vi "3458A Digitizing Process.vi"(8 "error in":errorcluster, 11 "session in":variant) -> (0 "error out":errorcluster, 3 "aux data out":variant)   [LabVIEW 2020, in "3458A Virtual Digitizer.lvlib"]
doc: "3458A digitizing lib: Main digitizing process. The VI is assynchronously executed once for each channel (all in parallel). It is started by calling 'Initiate Digitizing Process'. It then samples and sends the digitized data via queues to main process where the data are collected using 'Fetch Digitized Data'. Configuration of the execution is stored in 'session in' variable, execution control details are in 'session in->proc setup' cluster. Each instance of this VI has ID starting from 0 which identifies to which channel it belongs to."
uses:
  3458A Virtual Digitizer.lvlib
  3458A Digitizer Session.ctl
  3458A Virtual Channel Config.ctl
  Counter/Counter Session.ctl
  Counter/Counter Type.ctl
  AWG/AWG Session.ctl
  AWG/AWG Type.ctl
  AWG/CMI Clock Divider v2/CMI ckd2 Session.ctl
  AWG/CMI Clock Divider v2/CMI ckd2 Source Mode.ctl
  AWG/CMI Clock Divider v2/CMI ckd2 Divisor Mode.ctl
  AWG/CMI Sync V3/CMI Sync V3 session.ctl
  AWG/CMI Sync V3/Configure/CMI Sync V3 Reference Clock Source.ctl
  AWG/CMI Sync V3/Configure/CMI Sync V3 HV input Range.ctl
  AWG/CMI Sync V3/Configure/CMI Sync V3 Trigger Input Level.ctl
  AWG/CMI Sync V3/Configure/CMI Sync V3 Channel 1 Mode.ctl
  AWG/CMI Sync V3/Configure/CMI Sync V3 Channel Output Levels.ctl
  AWG/CMI Sync V3/Configure/CMI Sync V3 Channel 2 Mode.ctl
  AWG/CMI Sync V3/Configure/CMI Sync V3 Channel 3 Mode.ctl
  AWG/CMI Sync V3/Configure/CMI Sync V3 Channel 1 Divisor Entry Mode.ctl
  adc/ADC Trig Config.ctl
  adc/ADC Trig Mode Source.ctl
  adc/ADC Trig Slope.ctl
  adc/ADC Trig Coupling.ctl
  AWG/RaS HMF2500/HMF2500 Config.ctl
  3458A Sync Mode.ctl
  3458A Idn Mode.ctl
  3458A Digitizing Low Levels/Configure/Sampling Mode.ctl
  3458A Digitizing Process Options.ctl
  3458A Data Packet.ctl
  3458A Aux Record Data.ctl
  3458A Digitizing Low Levels/Configure/Level Setup.ctl
  3458A Digitizing Low Levels/Configure/First Sample Trigger.ctl
  3458A Aperture Selection Mode.ctl
  3458A Multiplexing Config.ctl
  Fluke 8588A/F8588A Low Pass Filter.ctl
  Fluke 8588A/F8588A Phase Lock.ctl
  Fluke 8588A/F8588A Coupling.ctl
  3458A Sampling Rate.ctl
  AWG/AWG Clock Setup Mode.ctl
  3458A Sample Rate Mode.ctl
  <vilib>/Utility/error.llb/Error Cluster From Error Code.vi
  <vilib>/ErrorRing/Error Ring.xnode
  Counter/Counter.lvlib
  AWG/AWG.lvlib
  3458A Digitizing Low Levels/3458A Digitizing Low Levels.lvlib
  3458A Basic Driver/3458A Basic Driver.lvlib
  AWG/CMI Sync V3/CMI Sync Unit V3.lvlib
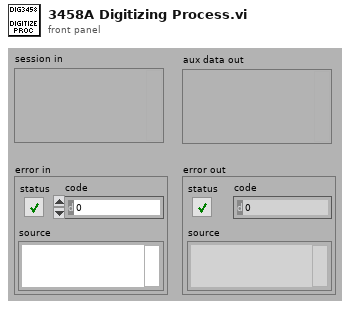
[diagram p1: front panel]
types:
  T1 = typedef "3458A Virtual Digitizer.lvlib/3458A Digitizing Low Levels.lvlib/First Sample Trigger.ctl" = enum16{"AUTO", "EXT", "SYN", "SGL", "HOLD", "LEVEL"}
  T2 = typedef "3458A Virtual Digitizer.lvlib/3458A Data Packet.ctl" = cluster{"data":i32[][], "offset [smpl]":i32, "count [smpl]":i32, "all done?":bool, "sampling?":bool, "queue buffer [%]":dbl, "valid?":bool, "overflow?":bool, "estimate info?":bool}
  T3 = typedef "3458A Virtual Digitizer.lvlib/3458A Digitizer Session.ctl" = cluster{"channels":T4[], "sync unit":T5, "awg unit":T7, "sync mode":T26, "streaming mode":bool, "idn mode":T27, "sampling mode":T28, "sample memory [B]":i32, "proc setup":T29, "sample size [B]":i32, "sample count":i32, "aux data":T31, "ranges [V]":dbl[], "aperture [s]":dbl, "LEVEL trigger":T32, "trigger mode":T1, "measure temp.?":bool, "disp mesages":string[], "shared bus?":bool, "disable display?":bool, "aper mode":T33, "aper rules":dbl[][], "multiplex":T34, "F8588 lpf":T35, "F8588 pll":T36, "F8588 couple":T37, "fs":T38, "fs mode":T40, "init timestamp":timestamp, "last report timestamp":timestamp}
  T4 = typedef "3458A Virtual Digitizer.lvlib/3458A Virtual Channel Config.ctl" = cluster{"VISA":refnum<visa-resource-name>, "Range [Vpk]":dbl, "btn clr":bool, "btn up":bool, "btn down":bool, "F8588":bool, "F8588 guard":bool}
  T5 = typedef "Counter.lvlib/Counter Session.ctl" = cluster{"VISA":refnum<visa-resource-name>, "type":T6}
  T6 = typedef "Counter.lvlib/Counter Type.ctl" = enum16{"Picotest U6200A", "dummy"}
  T7 = typedef "AWG.lvlib/AWG Session.ctl" = cluster{"type":T8, "VISA":refnum<visa-resource-name>, "enable 10MHz ref":bool, "cmi ckd2":T9, "cmi sync v3":T12, "trigger":T21, "HMF2500 cfg":T25}
  T8 = typedef "AWG.lvlib/AWG Type.ctl" = enum16{"Agilent 331xxA to 332xxA", "Agilent 335xxA to 336xxA", "Tektronix AFG3101C", "R&S HMF25xx", "CMI Clock Divider v2", "CMI Sync Unit V3", "dummy"}
  T9 = typedef "AWG.lvlib/CMI ckd2 Session.ctl" = cluster{"VISA":refnum<visa-resource-name>, "clock source":T10, "manual ref clk":bool, "ref clock [Hz]":dbl, "div mode":T11}
  T10 = typedef "AWG.lvlib/CMI ckd2 Source Mode.ctl" = enum16{"Auto", "LF clock", "HF clock", "Internal"}
  T11 = typedef "AWG.lvlib/CMI ckd2 Divisor Mode.ctl" = enum16{"Set divisor directly", "Set divisor by frequency"}
  T12 = typedef "AWG.lvlib/CMI Sync Unit V3.lvlib/CMI Sync V3 session.ctl" = cluster{"VISA":refnum<visa-resource-name>, "baud rate [bd/s]":i32, "source":T13, "hv range":T14, "fsrc is fixed":bool, "fsrc [Hz]":dbl, "freq integ [s]":dbl, "freq filter":i32, "trig level":T15, "chn1 mode":T16, "chn1 level":T17, "chn2 mode":T18, "chn2 level":T17, "chn2 div":i32, "chn3 mode":T19, "chn3 level":T17, "chn1 div entry":T20, "chn1 dev limit [%]":dbl, "chn1 check dev":bool}
  T13 = typedef "AWG.lvlib/CMI Sync Unit V3.lvlib/CMI Sync V3 Reference Clock Source.ctl" = enum16{"Auto", "Internal", "Logic", "Sine", "HV"}
  T14 = typedef "AWG.lvlib/CMI Sync Unit V3.lvlib/CMI Sync V3 HV input Range.ctl" = enum16{"10V", "60V", "250V", "1kV"}
  T15 = typedef "AWG.lvlib/CMI Sync Unit V3.lvlib/CMI Sync V3 Trigger Input Level.ctl" = enum16{"LVCMOS 3V3", "TTL 5V"}
  T16 = typedef "AWG.lvlib/CMI Sync Unit V3.lvlib/CMI Sync V3 Channel 1 Mode.ctl" = enum16{"Source divider", "DDS absolute", "DDS ratio", "DDS ratio M/N"}
  T17 = typedef "AWG.lvlib/CMI Sync Unit V3.lvlib/CMI Sync V3 Channel Output Levels.ctl" = enum16{"Positive 3V3", "Negative 3V3", "Positive 5V", "Negative 5V"}
  T18 = typedef "AWG.lvlib/CMI Sync Unit V3.lvlib/CMI Sync V3 Channel 2 Mode.ctl" = enum16{"Source divider", "Chn 1 divide"}
  T19 = typedef "AWG.lvlib/CMI Sync Unit V3.lvlib/CMI Sync V3 Channel 3 Mode.ctl" = enum16{"Chn 1 Active", "Chn 2 Active", "Chn 1 Trigger", "Chn 2 Trigger", "Gate", "PPS", "10MHz"}
  T20 = typedef "AWG.lvlib/CMI Sync Unit V3.lvlib/CMI Sync V3 Channel 1 Divisor Entry Mode.ctl" = enum16{"Set divisor directly", "Calculate nearest divisor from measured fx"}
  T21 = typedef "ADC Trig Config.ctl" = cluster{"source":T22, "slope":T23, "coupling":T24, "level [V]":dbl, "hysteresis [V]":dbl, "pre-trigger [%]":dbl}
  T22 = typedef "ADC Trig Mode Source.ctl" = enum16{"Immediate", "External", "Level"}
  T23 = typedef "ADC Trig Slope.ctl" = enum16{"POS", "NEG"}
  T24 = typedef "ADC Trig Coupling.ctl" = enum16{"DC", "AC"}
  T25 = typedef "AWG.lvlib/HMF2500 Config.ctl" = cluster{"Baud Rate":u32, "Parity":u16, "Data Bits":u16, "Flow Control":u16}
  T26 = typedef "3458A Virtual Digitizer.lvlib/3458A Sync Mode.ctl" = enum16{"MASTER-SLAVE, MASTER clocked by TIMER", "MASTER-SLAVE, MASTER clocked by AWG", "ALL clocked by AWG", "MASTER-SLAVE, ALL clocked by TIMER", "ALL clocked by AWG with DFLL"}
  T27 = typedef "3458A Virtual Digitizer.lvlib/3458A Idn Mode.ctl" = enum16{"Auto", "Sequential (chn A, chn B, ...)", "From calibration string"}
  T28 = typedef "3458A Virtual Digitizer.lvlib/3458A Digitizing Low Levels.lvlib/Sampling Mode.ctl" = enum16{"DCV", "DSDC", "DSAC"}
  T29 = typedef "3458A Virtual Digitizer.lvlib/3458A Digitizing Process Options.ctl" = cluster{"channel id":i32, "packet size [smpl]":i32, "current timeout [s]":dbl, "blk2blk timeout [s]":dbl, "event time":timestamp, "stop notifier":refnum<notifier>, "data queues":refnum<queue>[], "proc refs":refnum<vi>[], "bus semaphore":T30}
  T30 = typedef "Semaphore RefNum" = refnum<k1>
  T31 = typedef "3458A Virtual Digitizer.lvlib/3458A Aux Record Data.ctl" = cluster{"channel id":i32, "valid?":bool[], "gain [V]":dbl[], "timestamp [s]":dbl[], "Ts [s]":dbl, "abs timestamp":timestamp, "t [deg C]":dbl[], "multiplex timestamp [s]":dbl, "only multiplex?":bool, "multiplex smpl offset":i64, "overflow?":bool}
  T32 = typedef "3458A Virtual Digitizer.lvlib/3458A Digitizing Low Levels.lvlib/Level Setup.ctl" = cluster{"edge":enum16{"POS", "NEG"}, "level [V]":dbl, "coupling":enum16{"DC", "AC"}}
  T33 = typedef "3458A Virtual Digitizer.lvlib/3458A Aperture Selection Mode.ctl" = enum16{"Manual", "Maximum", "Table"}
  T34 = typedef "3458A Virtual Digitizer.lvlib/3458A Multiplexing Config.ctl" = cluster{"cycles":i32, "delay [s]":dbl, "enabled":bool, "overhead [s]":dbl, "tot smpls":i64, "sub-rec":i32, "overhead [%]":dbl, "emulated":bool}
  T35 = typedef "F8588A Low Pass Filter.ctl" = enum16{"Off", "100 kHz", "3 MHz"}
  T36 = typedef "F8588A Phase Lock.ctl" = enum16{"Off", "1 MHz", "10 MHz"}
  T37 = typedef "F8588A Coupling.ctl" = enum16{"AC, 1 MOhm", "AC, 10 MOhm", "DC, 1 MOhm", "DC, 10 MOhm", "DC, auto"}
  T38 = typedef "3458A Virtual Digitizer.lvlib/3458A Sampling Rate.ctl" = cluster{"freq mode":T39, "fs [Hz]":dbl, "fref [Hz]":dbl, "mul":dbl, "div":dbl}
  T39 = typedef "AWG.lvlib/AWG Clock Setup Mode.ctl" = enum16{"fs or Ts", "fs or Ts with fref", "fref/N", "fref*M/N", "fref*Ratio"}
  T40 = typedef "3458A Sample Rate Mode.ctl" = enum16{"fs or Ts", "fs*M/N"}
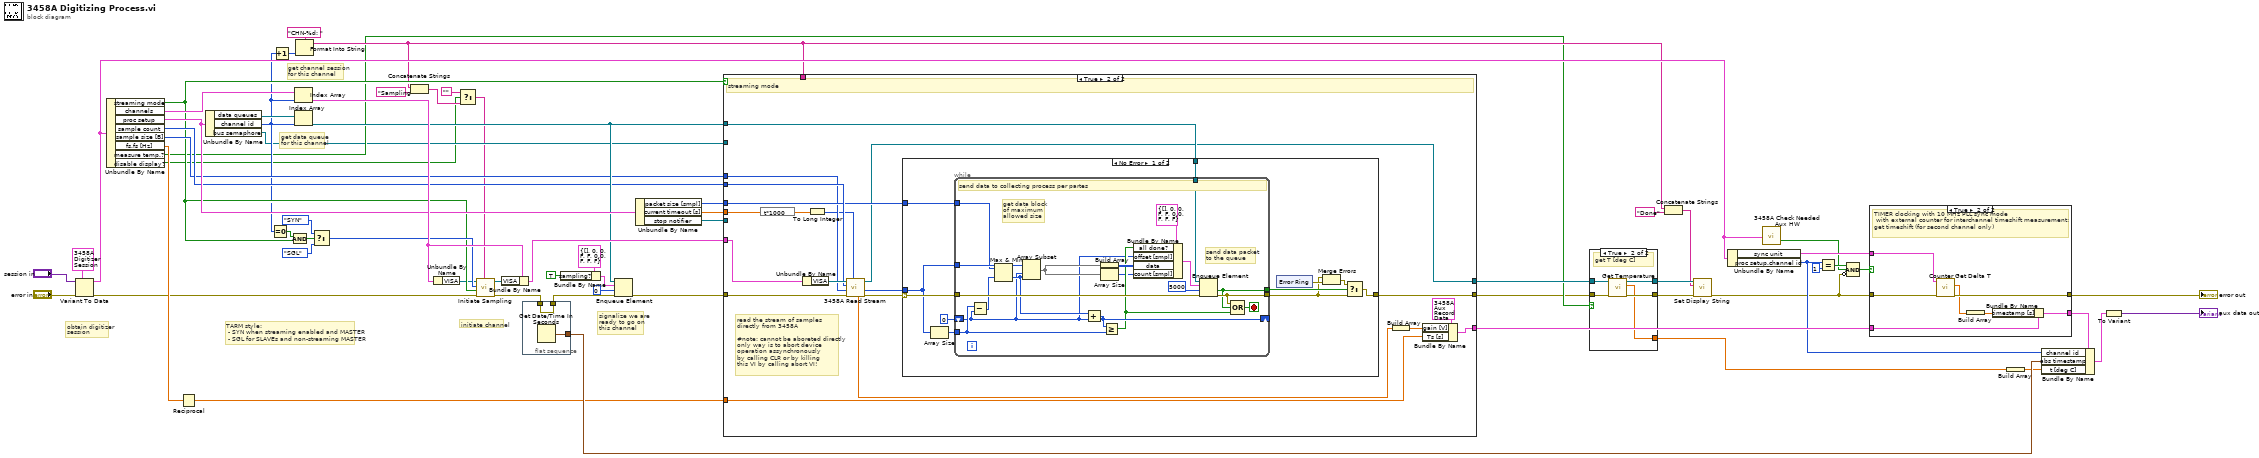
[diagram p0: block diagram]
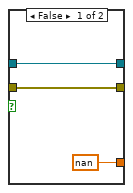
[diagram p2: hidden frame]
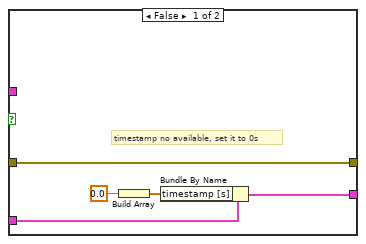
[diagram p3: hidden frame]
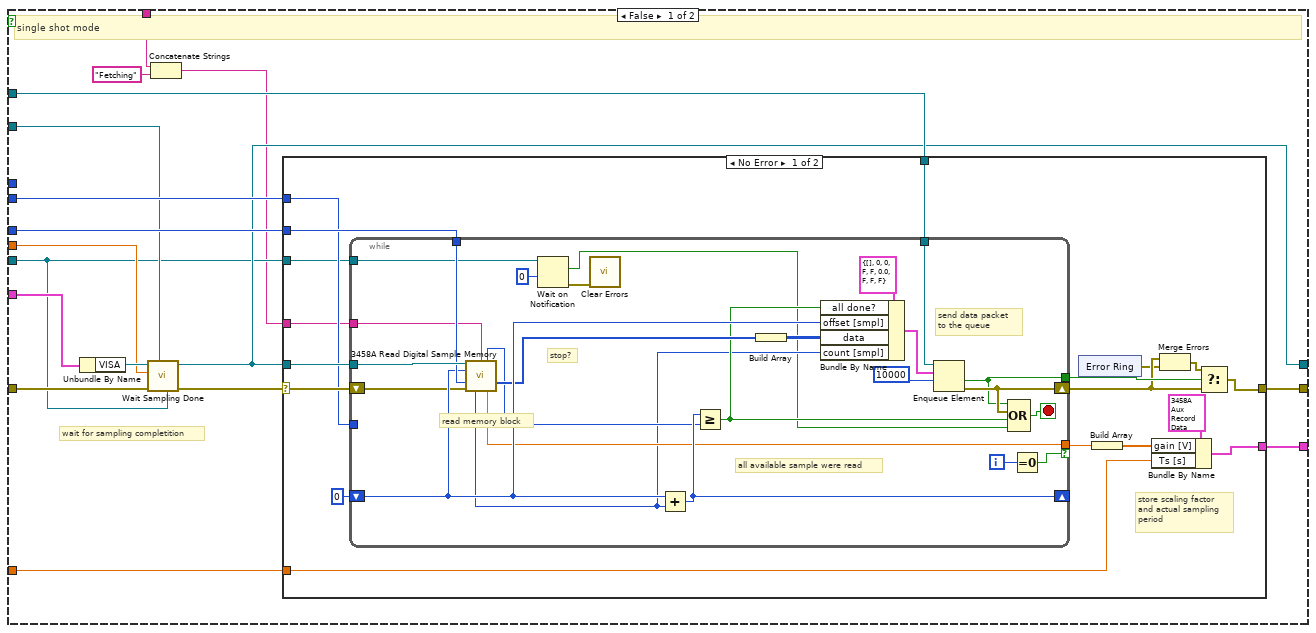
[diagram p4: hidden frame]
diagram:
  # "TARM style:\n - SYN when streaming enabled and MASTER\n - SGL for SLAVEs and non-streaming MASTER"
  # "get channel session\nfor this channel"
  # "get data queue\nfor this channel"
  # "signalize we are\nready to go on \nthis channel"
  # "initiate channel"
  # "obtain digitizer\nsession"
  n1 = Variant To Data(error in="error in", type=T3 {"channels"=[], "sync unit"={"VISA"="", "type"=enum."Picotest U6200A"}, "awg unit"={"type"=enum."Agilent 331xxA to 332xxA", "VISA"="", "enable 10MHz ref"=FALSE, "cmi ckd2"={"VISA"="", "clock source"=enum."Auto", "manual ref clk"=FALSE, "ref clock [Hz]"=0.0, "div mode"=enum."Set divisor directly"}, "cmi sync v3"={"VISA"="", "baud rate [bd/s]"=115200, "source"=enum."Auto", "hv range"=enum."1kV", "fsrc is fixed"=FALSE, "fsrc [Hz]"=10000000.0, "freq integ [s]"=1.0, "freq filter"=5, "trig level"=enum."TTL 5V", "chn1 mode"=enum."Source divider", "chn1 level"=enum."Positive 5V", "chn2 mode"=enum."Source divider", "chn2 level"=enum."Positive 5V", "chn2 div"=1, "chn3 mode"=enum."Chn 1 Active", "chn3 level"=enum."Positive 5V", "chn1 div entry"=enum."Calculate nearest divisor from measured fx", "chn1 dev limit [%]"=1.0, "chn1 check dev"=FALSE}, "trigger"={"source"=enum."Immediate", "slope"=enum."POS", "coupling"=enum."DC", "level [V]"=0.0, "hysteresis [V]"=0.0, "pre-trigger [%]"=0.0}, "HMF2500 cfg"={"Baud Rate"=9600, "Parity"=0, "Data Bits"=8, "Flow Control"=4}}, "sync mode"=enum."MASTER-SLAVE, MASTER clocked by TIMER", "streaming mode"=FALSE, "idn mode"=enum."Auto", "sampling mode"=enum."DCV", "sample memory [B]"=0, "proc setup"={"channel id"=0, "packet size [smpl]"=0, "current timeout [s]"=0.0, "blk2blk timeout [s]"=0.0, "event time"=timestamp(0 s since 1904-01-01), "stop notifier"=refnum, "data queues"=[], "proc refs"=[], "bus semaphore"=refnum}, "sample size [B]"=0, "sample count"=0, "aux data"={"channel id"=0, "valid?"=[], "gain [V]"=[], "timestamp [s]"=[], "Ts [s]"=0.0, "abs timestamp"=timestamp(0 s since 1904-01-01), "t [deg C]"=[], "multiplex timestamp [s]"=-1.0, "only multiplex?"=FALSE, "multiplex smpl offset"=0, "overflow?"=FALSE}, "ranges [V]"=[], "aperture [s]"=0.0, "LEVEL trigger"={"edge"=enum."POS", "level [V]"=0.0, "coupling"=enum."DC"}, "trigger mode"=enum."AUTO", "measure temp.?"=FALSE, "disp mesages"=[], "shared bus?"=FALSE, "disable display?"=FALSE, "aper mode"=enum."Manual", "aper rules"=[], "multiplex"={"cycles"=0, "delay [s]"=0.0, "enabled"=FALSE, "overhead [s]"=1.0, "tot smpls"=0, "sub-rec"=0, "overhead [%]"=0.0, "emulated"=FALSE}, "F8588 lpf"=enum."Off", "F8588 pll"=enum."Off", "F8588 couple"=enum."DC, auto", "fs"={"freq mode"=enum."fs or Ts", "fs [Hz]"=0.0, "fref [Hz]"=0.0, "mul"=0.0, "div"=0.0}, "fs mode"=enum."fs or Ts", "init timestamp"=timestamp(0 s since 1904-01-01), "last report timestamp"=timestamp(0 s since 1904-01-01)} ("digitizer session"), Variant="session in") -> (data=w43:T3, error out=w21:errorcluster)
  n2 = Unbundle By Name(w43) -> ("streaming mode"=w26:bool, "channels"=w63:T4[], "proc setup"=w55:T29, "sample count"=w50:i32, "sample size [B]"=w35:i32, "fs.fs [Hz]"=w30:dbl, "measure temp.?"=w10:bool, "disable display?"=w3:bool)
  n3 = Reciprocal(x=w30) -> (1/x=w1:dbl)
  n4 = Unbundle By Name(w55) -> ("data queues"=w62:refnum<queue>[], "channel id"=w17:i32, "bus semaphore"=w8:T30)
  n5 = Equal To 0?(x=w17) -> (x = 0?=w33:bool)
  n6 = Increment(x=w17) -> (x+1=w16:i32)
  n7 = Compound Arithmetic op=AND(w33, w26) -> (w34:bool)
  n8 = Index Array(array=w63, index=w17) -> (element=w61:T4)
  n9 = Index Array(array=w62, index=w17) -> (element=w51:refnum<queue>)
  n10 = Format Into String(format string="CHN-%d: ", w16) -> (resulting string=w11:string)  [unwired: 2 in, 1 out]
  n11 = Select(t=First_Sample_Trigger."SYN" ("ARM mode (SGL)"), s=w34, f=First_Sample_Trigger."SGL" ("ARM mode (SGL)")) -> (s? t:f=w27:T1)
  n12 = Concatenate Strings(w11, "Sampling" ("string")) -> (w4:string)
  n13 = Unbundle By Name(w61) -> ("VISA"=w20:refnum<visa-resource-name>)
  n14 = Select(t="", s=w3, f=w4) -> (s? t:f=w5:string)
  n15 = call "Initiate Sampling.vi"("display string (none)"=w5, "error in"=w21, "stream mode (False)"=w26, "ARM mode (SGL)"=w27, "VISA resource in"=w20) -> ("error out"=w29:errorcluster, "VISA resource out"=w36:refnum<visa-resource-name>)  [unwired: 5 in]
  n16 = Bundle By Name(cluster=w61, "VISA"=w36) -> (w56:T4)
  n17 = flat-sequence {
    tunnel: w29 -> [w67]
    tunnel: [w67] -> w28
    tunnel: [w66] -> w24
    frame #0 {
      n18 = Get Date/Time In Seconds() -> (seconds since 1Jan1904=w66:timestamp)
    }
  }
  n19 = Bundle By Name(cluster=T2 {"data"=[], "offset [smpl]"=0, "count [smpl]"=0, "all done?"=FALSE, "sampling?"=FALSE, "queue buffer [%]"=0.0, "valid?"=FALSE, "overflow?"=FALSE, "estimate info?"=FALSE} ("niScope packet"), "sampling?"=TRUE) -> (w58:T2)
  n20 = Enqueue Element(queue=w51, element=w58, timeout in ms (-1)=0, error in (no error)=w28) -> (error out=w37:errorcluster)  [unwired: 2 out]
  n21 = Unbundle By Name(w55) -> ("packet size [smpl]"=w52:i32, "current timeout [s]"=w54:dbl, "stop notifier"=w53:refnum<notifier>)
  n22 = case shown="True" w26 {
    tunnel: w37 -> [w76 w152]
    tunnel: w56 -> [w82 w151]
    tunnel: w54 -> [w83 w143]
    tunnel: w53 -> [w69 _]
    tunnel: w52 -> [w81 w140]
    tunnel: w51 -> [w80 w148]
    tunnel: w50 -> [w79 w149]
    tunnel: [w78 w139] -> w7
    tunnel: [w77 w146] -> w44
    tunnel: w35 -> [_ w138]
    tunnel: w1 -> [w75 w134]
    tunnel: [w71 w135] -> w25
    tunnel: w11 -> [w73 _]
    tunnel: w8 -> [w70 _]
    frame False {
      # "wait for sampling completition"
      # "single shot mode"
      n23 = Unbundle By Name(w82) -> ("VISA"=w84:refnum<visa-resource-name>)
      n24 = call "Wait Sampling Done.vi"("stop notifier ref (none)"=w69, "semaphore"=w70, "error in"=w76, "timeout [s] (5s)"=w83, "VISA resource in"=w84) -> ("error out"=w72:errorcluster, "VISA resource out"=w71:refnum<visa-resource-name>)  [unwired: 5 in]
      n25 = Concatenate Strings(w73, "Fetching" ("string")) -> (w68:string)
      n26 = case shown="No Error" w72 {
        selector: w72 -> [w101 w133]
        tunnel: w71 -> [w102 _]
        tunnel: w81 -> [w99 _]
        tunnel: w80 -> [w98 _]
        tunnel: w79 -> [w97 _]
        tunnel: [w91 w133] -> w78
        tunnel: [w94 _] -> w77
        tunnel: w75 -> [w87 _]
        tunnel: w68 -> [w86 _]
        tunnel: w69 -> [w85 _]
        frame No Error {
          # "store scaling factor\nand actual sampling\nperiod"
          n27 = while {
            tunnel: w102 -> [w129]
            shift-right: [w120] -> w89
            shift-left: w101 -> [w112]
            shift-right: [w124] -> _
            shift-left: 0 -> [w126]
            tunnel: w99 -> [w128]
            tunnel: w98 -> [w127]
            tunnel: w97 -> [_]
            tunnel: [w123] -> w95 if=w121
            tunnel: [w116] -> w92
            tunnel: w86 -> [w113]
            tunnel: w85 -> [w111]
            i -> [w122]
            stop <- w118 stop-if-true
            # "stop?"
            # "all available sample were read"
            # "read memory block"
            # "send data packet\nto the queue"
            n28 = call "3458A Read Digital Sample Memory.vi"("VISA session"=w129, "display string (none)"=w113, "First Read in Memory Location (0)"=w126, "max read [smpl]"=w128, "error in (no error)"=w112) -> ("total samples in memory?"=w115:i32, "waveform data int32"=w125:i32[], "read samples"=w114:i32, "scale factor"=w123:dbl)  [unwired: 4 in, 3 out]
            n29 = Wait on Notification(notifier=w111, timeout in ms (-1)=0) -> (notification=w108:bool, error out=w110:errorcluster)  [unwired: 2 in, 2 out]
            n30 = call <vilib>:"Clear Errors.vi"("error in (no error)"=w110) -> ()  [unwired: 5 in, 2 out]
            n31 = Add(x=w126, y=w114) -> (x+y=w124:i32)
            n32 = Greater Or Equal?(x=w124, y=w115) -> (x >= y?=w119:bool)
            n33 = Build Array(w125) -> (w117:i32[][])
            n34 = Bundle By Name(cluster=T2 {"data"=[], "offset [smpl]"=0, "count [smpl]"=0, "all done?"=FALSE, "sampling?"=FALSE, "queue buffer [%]"=0.0, "valid?"=FALSE, "overflow?"=FALSE, "estimate info?"=FALSE} ("niScope packet"), "all done?"=w119, "offset [smpl]"=w126, "data"=w117, "count [smpl]"=w114) -> (w131:T2)
            n35 = Enqueue Element(queue=w127, element=w131, timeout in ms (-1)=10000) -> (timed out?=w116:bool, error out=w120:errorcluster)  [unwired: 1 in, 1 out]
            n36 = Compound Arithmetic op=OR(w116, w120, w119, w108) -> (w118:bool)
            n37 = Equal To 0?(x=w122) -> (x = 0?=w121:bool)
          }
          n38 = xnode "Error Ring"() -> ("error out"=w88:errorcluster)
          n39 = Build Array(w95) -> (w93:dbl[])
          n40 = Bundle By Name(cluster=T31 {"channel id"=0, "valid?"=[], "gain [V]"=[], "timestamp [s]"=[], "Ts [s]"=0.0, "abs timestamp"=timestamp(0 s since 1904-01-01), "t [deg C]"=[], "multiplex timestamp [s]"=0.0, "only multiplex?"=FALSE, "multiplex smpl offset"=0, "overflow?"=FALSE} ("aux data"), "gain [V]"=w93, "Ts [s]"=w87) -> (w94:T31)
          n41 = Merge Errors(w89, w88) -> (w90:errorcluster)
          n42 = Select(t=w90, s=w92, f=w89) -> (s? t:f=w91:errorcluster)
        }
        frame Error {
          # "timeout occured, do nothing"
        }
      }
    }
    frame True {
      # "read the stream of samples\ndirectly from 3458A\n\n#note: cannot be aboreted directly\nonly way is to abort device\noperation assynchronously\nby calling CLR or by killing\nthis VI by calling abort VI!"
      # "streaming mode"
      n43 = expression code="t*1000"(w143) -> (w142:dbl)
      n44 = Unbundle By Name(w151) -> ("VISA"=w150:refnum<visa-resource-name>)
      n45 = To Long Integer(number=w142) -> (32bit integer=w136:i32)
      n46 = call "3458A Read Stream.vi"("read timeout [ms] (30000s)"=w136, "error in (no error)"=w152, "sample size [B]"=w138, "samples count"=w149, "VISA session"=w150) -> ("error out"=w137:errorcluster, "waveform data int32"=w141:i32[], "dup VISA session"=w135:refnum<visa-resource-name>, "scale factor"=w145:dbl)  [unwired: 1 in, 2 out]
      n47 = case shown="No Error" w137 {
        selector: w137 -> [w156 w188]
        tunnel: w148 -> [w163 _]
        tunnel: w141 -> [w153 _]
        tunnel: w140 -> [w161 _]
        tunnel: [w157 w188] -> w139
        frame No Error {
          n48 = Array Size(array=w153) -> (size(s)=w155:i32)
          n49 = while {
            tunnel: w156 -> [w184]
            tunnel: [w179] -> w154
            tunnel: w163 -> [w183]
            tunnel: w153 -> [w181]
            shift-right: [w180] -> _
            shift-left: 0 -> [w169]
            tunnel: w161 -> [w175]
            tunnel: w155 -> [w176]
            tunnel: [w177] -> w158
            stop <- w178 stop-if-true
            # "get data block\nof maximum\nallowed size"
            # "send data packet\nto the queue"
            # "send data to collecting process per partes"
            n50 = Subtract(x=w176, y=w169) -> (x-y=w174:i32)
            n51 = Max & Min(x=w175, y=w174) -> (min(x,y)=w173:i32)  [unwired: 1 out]
            n52 = Array Subset(array=w181, index=w169, length=w173) -> (w170:i32[])
            n53 = Add(x=w173, y=w169) -> (x+y=w180:i32)
            n54 = Build Array(w170) -> (w182:i32[][])
            n55 = Array Size(array=w170) -> (size(s)=w171:i32)
            n56 = Greater Or Equal?(x=w180, y=w176) -> (x >= y?=w172:bool)
            n57 = Bundle By Name(cluster=T2 {"data"=[], "offset [smpl]"=0, "count [smpl]"=0, "all done?"=FALSE, "sampling?"=FALSE, "queue buffer [%]"=0.0, "valid?"=FALSE, "overflow?"=FALSE, "estimate info?"=FALSE} ("niScope packet"), "all done?"=w172, "offset [smpl]"=w169, "data"=w182, "count [smpl]"=w171) -> (w186:T2)
            n58 = Enqueue Element(queue=w183, element=w186, timeout in ms (-1)=5000, error in (no error)=w184) -> (timed out?=w177:bool, error out=w179:errorcluster)  [unwired: 1 out]
            n59 = Compound Arithmetic op=OR(w179, w177, w172) -> (w178:bool)
          }
          n60 = xnode "Error Ring"() -> ("error out"=w159:errorcluster)
          n61 = Merge Errors(w154, w159) -> (w160:errorcluster)
          n62 = Select(t=w160, s=w158, f=w154) -> (s? t:f=w157:errorcluster)
        }
        frame Error {
        }
      }
      n63 = Build Array(w145) -> (w147:dbl[])
      n64 = Bundle By Name(cluster=T31 {"channel id"=0, "valid?"=[], "gain [V]"=[], "timestamp [s]"=[], "Ts [s]"=0.0, "abs timestamp"=timestamp(0 s since 1904-01-01), "t [deg C]"=[], "multiplex timestamp [s]"=0.0, "only multiplex?"=FALSE, "multiplex smpl offset"=0, "overflow?"=FALSE} ("aux data"), "gain [V]"=w147, "Ts [s]"=w134) -> (w146:T31)
    }
  }
  n65 = case shown="True" w10 {
    tunnel: w7 -> [w190 w196]
    tunnel: [w190 w195] -> w19
    tunnel: [w191 w194] -> w18
    tunnel: w25 -> [w191 w193]
    tunnel: [nan w192] -> w23
    frame False {
    }
    frame True {
      # "get T [deg C]"
      n66 = call "Get Temperature.vi"("error in(no error)"=w196, "VISA Resource Name"=w193) -> ("error out"=w195:errorcluster, "temperature [deg C]"=w192:dbl, "VISA resource name out"=w194:refnum<visa-resource-name>)  [unwired: 7 in]
    }
  }
  n67 = Concatenate Strings(w11, "Done" ("string")) -> (w13:string)
  n68 = call "Set Display String.vi"("error in(no error)"=w19, "display string (none)"=w13, "VISA Resource Name"=w18) -> ("error out"=w6:errorcluster)  [unwired: 7 in, 1 out]
  n69 = Unbundle By Name(w43) -> ("sync unit"=w47:T5, "proc setup.channel id"=w38:i32)
  n70 = call "3458A Check Needed Aux HW.vi"("digitizer session"=w43) -> ("uses counter for delta T sync?"=w42:bool)  [unwired: 13 in, 5 out]
  n71 = Equal?(x=w38, y=1) -> (x = y?=w45:bool)
  n72 = Compound Arithmetic op=AND(w45, w42, invert w6) -> (w48:bool)
  n73 = case shown="True" w48 {
    tunnel: w6 -> [w201 w205]
    tunnel: w47 -> [_ w203]
    tunnel: w44 -> [w199 w208]
    tunnel: [w201 w204] -> w9
    tunnel: [w200 w207] -> w39
    frame False {
      # "timestamp no available, set it to 0s"
      n74 = Build Array(0.0 ("time stamp [s]")) -> (w198:dbl[])
      n75 = Bundle By Name(cluster=w199, "timestamp [s]"=w198) -> (w200:T31)
    }
    frame True {
      # "TIMER clocking with 10 MHz PLL sync mode\n with external counter for interchannel timeshift measurement:\nget timeshift (for second channel only)"
      n76 = call "Counter Get Delta T.vi"("error in"=w205, "counter session in"=w203) -> ("error out"=w204:errorcluster, "delta t [s]"=w202:dbl)  [unwired: 7 in, 1 out]
      n77 = Build Array(w202) -> (w206:dbl[])
      n78 = Bundle By Name(cluster=w208, "timestamp [s]"=w206) -> (w207:T31)
    }
  }
  "error out" <- w9
  n79 = Build Array(w23) -> (w22:dbl[])
  n80 = Bundle By Name(cluster=w39, "channel id"=w38, "abs timestamp"=w24, "t [deg C]"=w22) -> (w40:T31)
  n81 = To Variant(anything=w40) -> (Variant=→"aux data out":variant)
